vi "My Traffic Light.vi"() -> ()   [LabVIEW 2020]
uses:
  OneDrive/Desktop/Work/labview exercises/stop_light_colors.ctl
panel:
  in  "stop":bool
  out "Red Light":bool
  out "Yellow Light":bool
  out "Green Light":bool
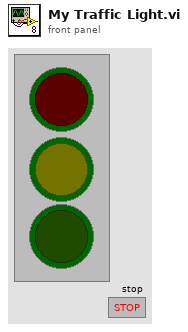
[diagram p1: front panel]
types:
  T1 = typedef "stop_light_colors.ctl" = enum16{"green", "yellow", "red"}
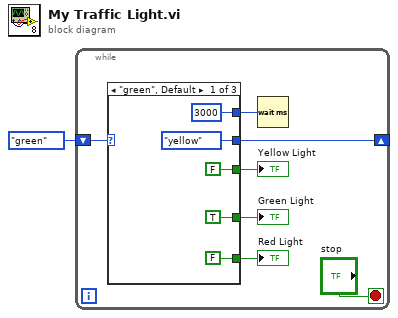
[diagram p0: block diagram]
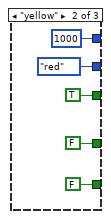
[diagram p2: hidden frame]
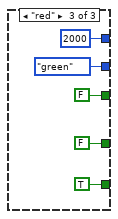
[diagram p3: hidden frame]
diagram:
  n1 = while {
    shift-right: [w7] -> _
    shift-left: stop_light_colors."green" -> [w8]
    stop <- "stop" stop-if-true
    n2 = case shown="\"green\", Default" w8 {
      tunnel: [stop_light_colors."yellow" stop_light_colors."red" stop_light_colors."green"] -> w7
      tunnel: [3000 1000 2000] -> w3
      tunnel: [FALSE FALSE TRUE] -> w6
      tunnel: [FALSE TRUE FALSE] -> w5
      tunnel: [TRUE FALSE FALSE] -> w4
      frame "green", Default {
      }
      frame "yellow" {
      }
      frame "red" {
      }
    }
    "Yellow Light" <- w5
    "Red Light" <- w6
    "Green Light" <- w4
    n3 = Wait (ms)(milliseconds to wait=w3) -> ()  [unwired: 1 out]
  }
